vi "MU Activate Calibration Config.vi"(8 "error in (no error)":errorcluster, 11 "MUhandle":u64) -> (0 "error out":errorcluster, 3 "function return":u32)   [LabVIEW 2017, in "MU_3SL_interface.lvlib"]
doc: "MU_PUBLIC MU_Error MU_activateCalibrationConfiguration(MU_Handle handle);"
uses:
  MU_3SL_interface.lvlib
  lib/MU_3SL_interface.dll
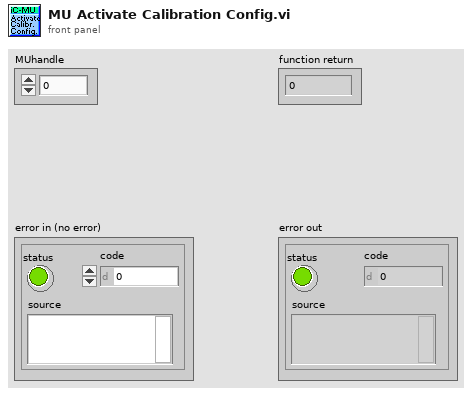
[diagram p1: front panel]
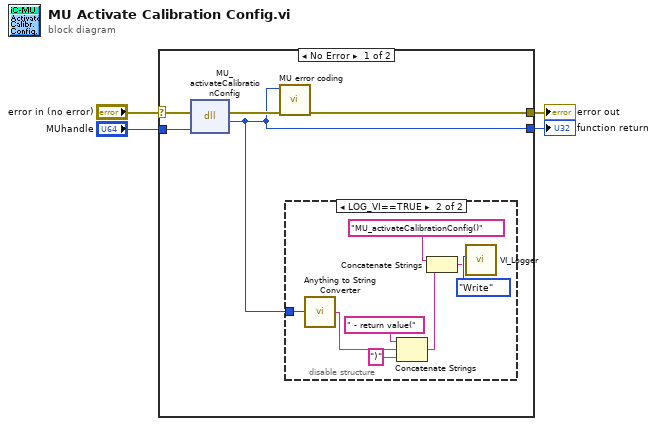
[diagram p0: block diagram]
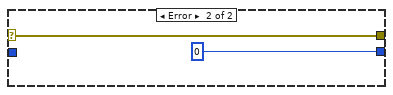
[diagram p3: hidden frame]
diagram:
  n1 = case shown="No Error" "error in (no error)" {
    selector: "error in (no error)" -> [w7 w19]
    tunnel: [w5 u32 0] -> w4
    tunnel: [w8 w19] -> w3
    tunnel: "MUhandle" -> [w6 _]
    frame No Error {
      n2 = dll-call lib="C:/Users/bes/AppData/Roaming/work/mu_9so/icsubmodules/soft_mu_3sl_master/lv_interface/lib/MU_3SL_interface**.*" fn="MU_activateCalibrationConfig"(error in=w7, "handle"=w6) -> (error out=w9:errorcluster, "return type"=w5:u32)  [unwired: 3 in, 1 out]
      n3 = call "MU error coding.vi"("error in (no error)"=w9, "function return in"=w5) -> ("error out"=w8:errorcluster)  [unwired: 9 in]
      n4 = disable-structure shown="LOG_VI==TRUE" {
        disable-tunnel: w5 -> [_ w11]
        frame condition #0 {
        }
        frame condition #1 (active) {
          n5 = call "Anything to String Converter.vi"("anything"=w11) -> ("String"=w10:string)
          n6 = Concatenate Strings(" - return value(" ("string"), w10, ")" ("string")) -> (w15:string)
          n7 = Concatenate Strings("MU_activateCalibrationConfig()" ("Info in"), w15) -> (w14:string)
          n8 = call "VI_Logger.vi"("Action (Read)"=enum16{"Write", "Read"}."Write", "Info in"=w14) -> ()  [unwired: 8 in, 2 out]
        }
      }
    }
    frame Error {
    }
  }
  "function return" <- w4
  "error out" <- w3
